vi "Write Grid Colors.vi"(5 "Grid Colors":cluster{"Major Color":u32, "Minor Color":u32}, 9 "GraphScale in":refnum<class "GraphScale.lvclass">) -> (3 "GraphScale out":refnum<class "GraphScale.lvclass">)   [LabVIEW 2014, in "Raspberry Pi Compatible Compiler for LabVIEW.lvlib" / "GraphScale.lvclass"]
uses:
  GraphScale.lvclass
  GraphScale.lvclass/GraphScale.ctl
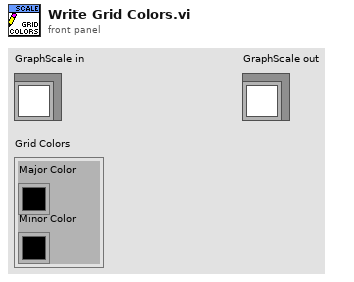
[diagram p1: front panel]
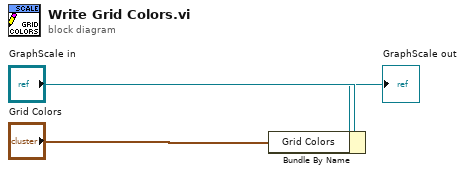
[diagram p0: block diagram]
diagram:
  n1 = Bundle By Name(cluster="GraphScale in", "Grid Colors"="Grid Colors") -> (→"GraphScale out":refnum<class "GraphScale.lvclass">)
